vi "output.vi"(8 "error in":errorcluster, 10 "data table in":T1, 11 "Engine to Engine Communication runtime in":refnum<class "E2E Runtime (RT FIFO).lvclass">) -> (0 "error out":errorcluster, 2 "data table out":T1, 3 "Engine to Engine Communication runtime out":refnum<class "E2E Runtime (RT FIFO).lvclass">)   [LabVIEW 2015, in "E2E Runtime (RT FIFO).lvclass"]
doc: "Provides an interface for writing data to a module at runtime. While this interface performs no operations, a child should provide an override which may write to any open sessions, references, or interfaces."
uses:
  E2E Runtime (RT FIFO).lvclass
  <vilib>/NI/Tag Bus/table/data table.ctl
  E2E Runtime (RT FIFO).lvclass/E2E Runtime (RT FIFO).ctl
  <vilib>/NI/Tag Bus/table/data polymorphs/read all/read all Doubles.vi
  <vilib>/NI/Tag Bus/table/data polymorphs/read all/read all Singles.vi
  <vilib>/NI/Tag Bus/table/data polymorphs/read all/read all I64s.vi
  <vilib>/NI/Tag Bus/table/data polymorphs/read all/read all I32s.vi
  <vilib>/NI/Tag Bus/table/data polymorphs/read all/read all I16s.vi
  <vilib>/NI/Tag Bus/table/data polymorphs/read all/read all I8s.vi
  <vilib>/NI/Tag Bus/table/data polymorphs/read all/read all U64s.vi
  <vilib>/NI/Tag Bus/table/data polymorphs/read all/read all U32s.vi
  <vilib>/NI/Tag Bus/table/data polymorphs/read all/read all U16s.vi
  <vilib>/NI/Tag Bus/table/data polymorphs/read all/read all U8s.vi
  <vilib>/NI/Tag Bus/table/data polymorphs/read all/read all Booleans.vi
  <vilib>/NI/Tag Bus/table/data table.lvlib
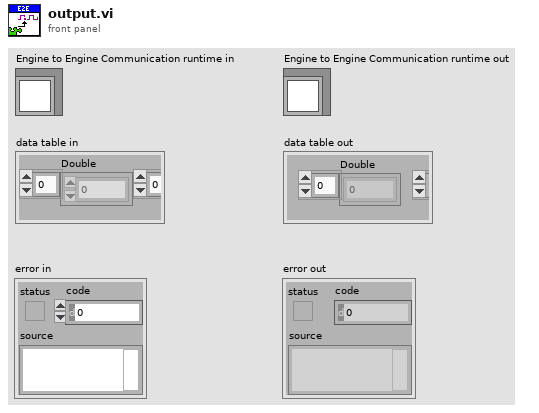
[diagram p1: front panel]
types:
  T1 = typedef "tag bus.lvlib/data table.lvlib/data table.ctl" = cluster{"Double":dbl[], "Single":sgl[], "I64":i64[], "I32":i32[], "I16":i16[], "I8":i8[], "U64":u64[], "U32":u32[], "U16":u16[], "U8":u8[], "Boolean":bool[], "String":string[], "Array of Double":cluster{"DBL Array":dbl[]}[], "Array of Single":cluster{"SGL Array":sgl[]}[], "Array of I64":cluster{"I64 Array":i64[]}[], "Array of I32":cluster{"I32 Array":i32[]}[], "Array of I16":cluster{"I16 Array":i16[]}[], "Array of I8":cluster{"I8 Array":i8[]}[], "Array of U64":cluster{"U64 Array":u64[]}[], "Array of U32":cluster{"U32 Array":u32[]}[], "Array of U16":cluster{"U16 Array":u16[]}[], "Array of U8":cluster{"U8 Array":u8[]}[], "Array of Boolean":cluster{"Boolean Array":bool[]}[], "Array of String":cluster{"String Array":string[]}[]}
  T2 = typedef "tag bus.lvlib/tag descriptor.lvclass/Data Type.ctl" = enum16{"Double", "Single", "I64", "I32", "I16", "I8", "U64", "U32", "U16", "U8", "Boolean", "String", "Array of Double", "Array of Single", "Array of I64", "Array of I32", "Array of I16", "Array of I8", "Array of U64", "Array of U32", "Array of U16", "Array of U8", "Array of Boolean", "Array of String"}
  T3 = typedef "E2E Runtime (RT FIFO).lvclass/Data FIFOs.ctl" = cluster{"Double":refnum<k33>, "Single":refnum<k33>, "I64":refnum<k33>, "I32":refnum<k33>, "I16":refnum<k33>, "I8":refnum<k33>, "U64":refnum<k33>, "U32":refnum<k33>, "U16":refnum<k33>, "U8":refnum<k33>, "Boolean":refnum<k33>}
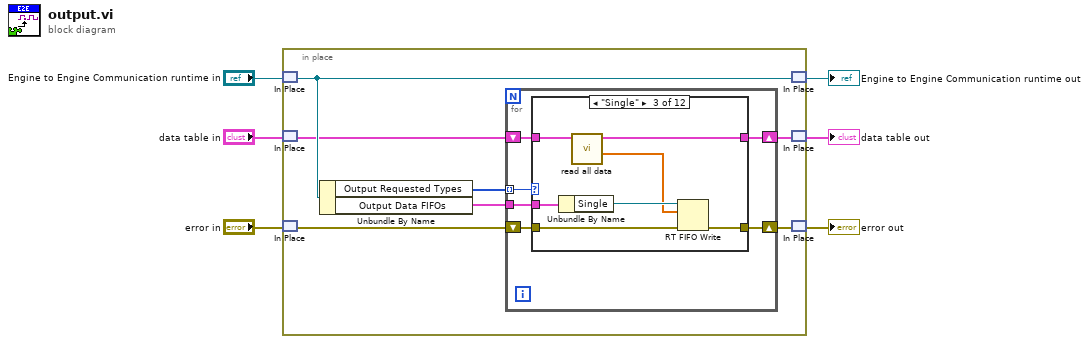
[diagram p0: block diagram]
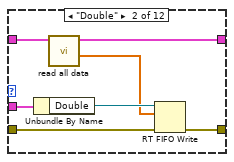
[diagram p3: hidden frame]
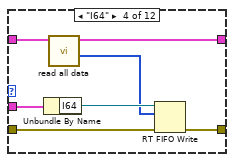
[diagram p4: hidden frame]
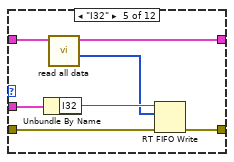
[diagram p5: hidden frame]
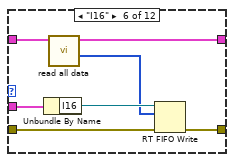
[diagram p6: hidden frame]
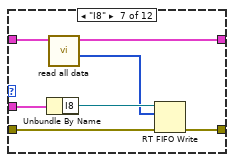
[diagram p7: hidden frame]
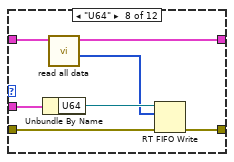
[diagram p8: hidden frame]
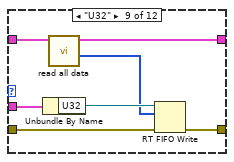
[diagram p9: hidden frame]
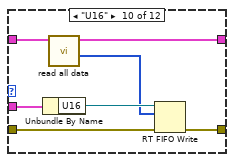
[diagram p10: hidden frame]
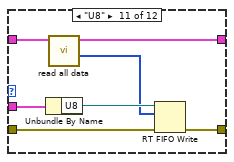
[diagram p11: hidden frame]
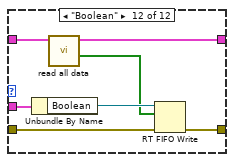
[diagram p12: hidden frame]
diagram:
  n1 = in-place {
    n2 = in-place-match #1("Engine to Engine Communication runtime in") -> (w13:refnum<class "E2E Runtime (RT FIFO).lvclass">)
    n3 = in-place-match #2("data table in") -> (w12:T1)
    n4 = in-place-match #3("error in") -> (w9:errorcluster)
    n5 = Unbundle By Name(w13) -> ("Output Requested Types"=w11:T2[], "Output Data FIFOs"=w10:T3)
    n6 = for {
      tunnel: w11 -> [w19] mode=indexing
      tunnel: w10 -> [w18]
      shift-right: [w15] -> w7
      shift-left: w9 -> [w17]
      shift-right: [w14] -> w8
      shift-left: w12 -> [w16]
      n7 = case shown="\"Single\"" w19 {
        tunnel: w18 -> [_ w28 w35 w42 w49 w56 w63 w70 w77 w84 w91 w98]
        tunnel: w17 -> [w21 w24 w31 w38 w45 w52 w59 w66 w73 w80 w87 w94]
        tunnel: w16 -> [w20 w27 w34 w41 w48 w55 w62 w69 w76 w83 w90 w97]
        tunnel: [w21 w22 w29 w36 w43 w50 w57 w64 w71 w78 w85 w92] -> w15
        tunnel: [w20 w26 w33 w40 w47 w54 w61 w68 w75 w82 w89 w96] -> w14
        frame Default {
        }
        frame "Double" {
          n8 = Unbundle By Name(w28) -> ("Double"=w25:refnum<k33>)
          n9 = call-poly <vilib>:"read all data.vi"("data table in"=w27) -> ("values"=w23:dbl[], "data table out"=w26:T1)  [unwired: 9 in]
          n10 = RT FIFO Write(0:w25, 1:w23, 3:w24) -> (11:w22:errorcluster)  [unwired: 2 in, 3 out]
        }
        frame "Single" {
          n11 = Unbundle By Name(w35) -> ("Single"=w32:refnum<k33>)
          n12 = call-poly <vilib>:"read all data.vi"("data table in"=w34) -> ("values"=w30:sgl[], "data table out"=w33:T1)  [unwired: 9 in]
          n13 = RT FIFO Write(0:w32, 1:w30, 3:w31) -> (11:w29:errorcluster)  [unwired: 2 in, 3 out]
        }
        frame "I64" {
          n14 = Unbundle By Name(w42) -> ("I64"=w39:refnum<k33>)
          n15 = call-poly <vilib>:"read all data.vi"("data table in"=w41) -> ("values"=w37:i64[], "data table out"=w40:T1)  [unwired: 9 in]
          n16 = RT FIFO Write(0:w39, 1:w37, 3:w38) -> (11:w36:errorcluster)  [unwired: 2 in, 3 out]
        }
        frame "I32" {
          n17 = Unbundle By Name(w49) -> ("I32"=w46:refnum<k33>)
          n18 = call-poly <vilib>:"read all data.vi"("data table in"=w48) -> ("values"=w44:i32[], "data table out"=w47:T1)  [unwired: 9 in]
          n19 = RT FIFO Write(0:w46, 1:w44, 3:w45) -> (11:w43:errorcluster)  [unwired: 2 in, 3 out]
        }
        frame "I16" {
          n20 = Unbundle By Name(w56) -> ("I16"=w53:refnum<k33>)
          n21 = call-poly <vilib>:"read all data.vi"("data table in"=w55) -> ("values"=w51:i16[], "data table out"=w54:T1)  [unwired: 9 in]
          n22 = RT FIFO Write(0:w53, 1:w51, 3:w52) -> (11:w50:errorcluster)  [unwired: 2 in, 3 out]
        }
        frame "I8" {
          n23 = Unbundle By Name(w63) -> ("I8"=w60:refnum<k33>)
          n24 = call-poly <vilib>:"read all data.vi"("data table in"=w62) -> ("values"=w58:i8[], "data table out"=w61:T1)  [unwired: 9 in]
          n25 = RT FIFO Write(0:w60, 1:w58, 3:w59) -> (11:w57:errorcluster)  [unwired: 2 in, 3 out]
        }
        frame "U64" {
          n26 = Unbundle By Name(w70) -> ("U64"=w67:refnum<k33>)
          n27 = call-poly <vilib>:"read all data.vi"("data table in"=w69) -> ("values"=w65:u64[], "data table out"=w68:T1)  [unwired: 9 in]
          n28 = RT FIFO Write(0:w67, 1:w65, 3:w66) -> (11:w64:errorcluster)  [unwired: 2 in, 3 out]
        }
        frame "U32" {
          n29 = Unbundle By Name(w77) -> ("U32"=w74:refnum<k33>)
          n30 = call-poly <vilib>:"read all data.vi"("data table in"=w76) -> ("values"=w72:u32[], "data table out"=w75:T1)  [unwired: 9 in]
          n31 = RT FIFO Write(0:w74, 1:w72, 3:w73) -> (11:w71:errorcluster)  [unwired: 2 in, 3 out]
        }
        frame "U16" {
          n32 = Unbundle By Name(w84) -> ("U16"=w81:refnum<k33>)
          n33 = call-poly <vilib>:"read all data.vi"("data table in"=w83) -> ("values"=w79:u16[], "data table out"=w82:T1)  [unwired: 9 in]
          n34 = RT FIFO Write(0:w81, 1:w79, 3:w80) -> (11:w78:errorcluster)  [unwired: 2 in, 3 out]
        }
        frame "U8" {
          n35 = Unbundle By Name(w91) -> ("U8"=w88:refnum<k33>)
          n36 = call-poly <vilib>:"read all data.vi"("data table in"=w90) -> ("values"=w86:u8[], "data table out"=w89:T1)  [unwired: 9 in]
          n37 = RT FIFO Write(0:w88, 1:w86, 3:w87) -> (11:w85:errorcluster)  [unwired: 2 in, 3 out]
        }
        frame "Boolean" {
          n38 = Unbundle By Name(w98) -> ("Boolean"=w95:refnum<k33>)
          n39 = call-poly <vilib>:"read all data.vi"("data table in"=w97) -> ("values"=w93:bool[], "data table out"=w96:T1)  [unwired: 9 in]
          n40 = RT FIFO Write(0:w95, 1:w93, 3:w94) -> (11:w92:errorcluster)  [unwired: 2 in, 3 out]
        }
      }
    }
    n41 = in-place-match #1(w13) -> (→"Engine to Engine Communication runtime out":refnum<class "E2E Runtime (RT FIFO).lvclass">)
    n42 = in-place-match #2(w8) -> (→"data table out":T1)
    n43 = in-place-match #3(w7) -> (→"error out":errorcluster)
  }
